vi "block message tester.vi"() -> ()   [LabVIEW 2020]
uses:
  Coherent Control/Type defs/Commands List.ctl
  Coherent Control/Type defs/Coherent commands direct mode.ctl
panel:
  out "trimmed string":string
  out "Response Validated ?":bool
  out "Response String":string
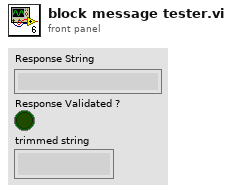
[diagram p1: front panel]
types:
  T1 = typedef "Coherent commands direct mode.ctl" = cluster{"Commands & Queries":T2, "Data String":string}
  T2 = typedef "Commands List.ctl" = enum16{"E", "B", "FL", "HM", "L", "LBOH", "LBOOPT", "LFP", "PROMPT", "SM", "S", "VW", "VWS", "HB", "HBR", "REQ", "ALIGN", "K", "F", "FH", "UF", "PHLDC", "PZTMC", "PZTXC", "PZTYC", "PHLDP", "PZTMP", "PZTXP", "PZTYP", "PTRK", "MDLK", "PP", "TS", "STPRPOS", "C", "D1C", "D2C", "BT", "D1T", "D2T", "VT", "LBOT", "ET", "D1ST", "D2ST", "VST", "LBOST", "EST", "D1TD", "D2TD", "VD", "LBOD", "ED", "D1HST", "D2HST", "LRS", "D1SS", "D2SS", "VSS", "LBOSS", "ESS", "D1H", "D2H", "HH", "D1V", "D2V", "SV", "MB", "PI", "BV", "AMDLK", "PZTS", "TMAX", "TMIN", "ALIGNP", "ALIGNW", "PZTXCM", "PZTXCP", "PZTXPM", "PZTXPP", "PZTYCM", "PZTYCP", "PZTYPM", "PZTYPP", "RH", "SN", "ST", "GDDCURVE", "GDD", "GDDCURVEN", "SETCURVEN", "SETCURVEPT", "SAVECURVE", "DELCURVE", "CURVEN", "CURVEPT", "CURVE", "COMP", "HMCOMP", "GDDMAX", "GDDMIN"}
  T3 = enum16{"Initialise", "Get Command", "Set Command", "Close"}
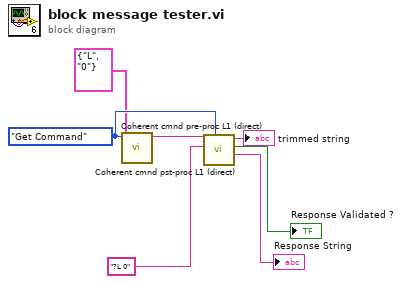
[diagram p0: block diagram]
diagram:
  w7 = T3."Get Command" ("Coherent laser commands L1")
  n1 = call "Coherent cmnd pre-proc L1 (direct).vi"("Coherent Commands"=T1 {"Commands & Queries"=enum."L", "Data String"="0"}, "Coherent laser commands L1"=w7) -> ("concatenated string"=w6:string)  [unwired: 9 in]
  n2 = call "Coherent cmnd pst-proc L1 (direct).vi"("Coherent laser commands L1"=w7, "Response String"="?L 0", "Command String"=w6) -> ("Response String"=→"Response String":string, "Response Validated ?"=→"Response Validated ?":bool, "trimmed string"=→"trimmed string":string)  [unwired: 4 in, 2 out]
